vi "t_KCubeActionEngine(V4).vi"(4 "SerialNumber":string="26004283", 5 "Motors // Simulate":bool, 6 "ChannelNumber":i32, 7 "Settings":T1={"Step Size (mm)"=10.0, "Step Delay (ms)"=0, "Velocity (mm/s)"=0.0, "Acceleration (mm/s^2)"=0.0} {"Step Size (mm)" min=0.00046 format="%.8f"}, 8 "error in":errorcluster, 9 "KCubeStepperControl":refnum<k24>(container), 10 "Action":T2, 11 "Input Position":dbl) -> (0 "error out":errorcluster, 1 "KCubeStepperControl Out":refnum<k24>, 2 "IsSettingsInitialized":bool, 3 "Current Position":dbl)   [LabVIEW 2022 SP3]
uses:
  C:/Users/mnopl/Desktop/Software/mnOPSuite/PRISM/Thorlabs.MotionControl.Controls.dll
  PRISM/Thorlabs.MotionControl.Controls.dll
  ActionEngineEnum(V2).ctl
  C:/Users/mnopl/Desktop/Software/mnOPSuite/PRISM/Thorlabs.MotionControl.KCube.StepperMotorCLI.dll
  PRISM/Thorlabs.MotionControl.KCube.StepperMotorCLI.dll
panel:
  in  "Value":dbl
  out "Simulation Status":string="Connection Open"
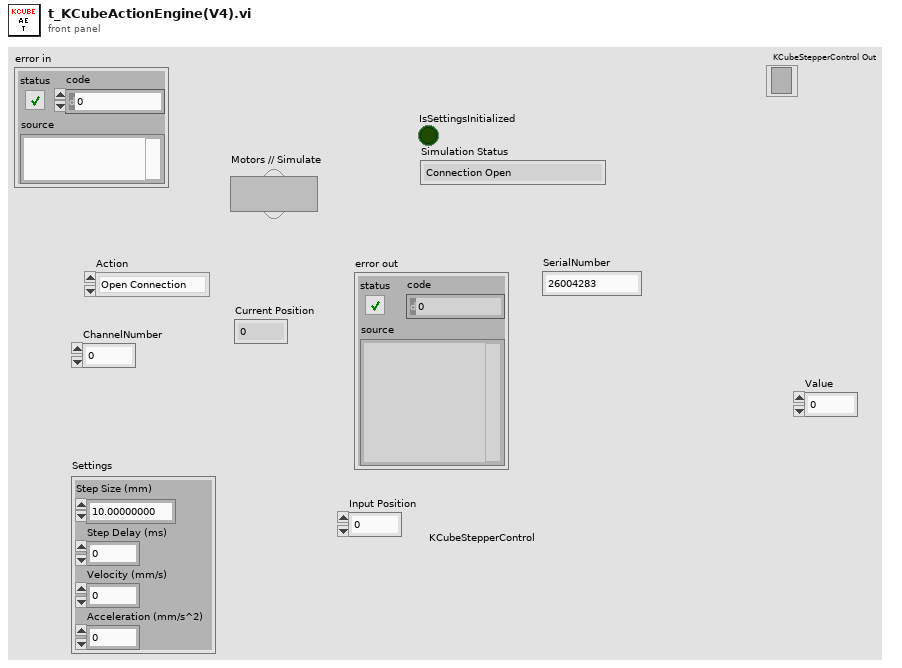
[diagram p1: front panel]
types:
  T1 = cluster{"Step Size (mm)":sgl, "Step Delay (ms)":u32, "Velocity (mm/s)":dbl, "Acceleration (mm/s^2)":dbl}
  T2 = typedef "ActionEngineEnum(V2).ctl" = enum16{"Open Connection", "IsSettingsInitialized? ", "Done", "Get Position", "Settings", "Home", "Move Absolute", "Move Relative", "Step", "Stop Action", "Close Connection"}
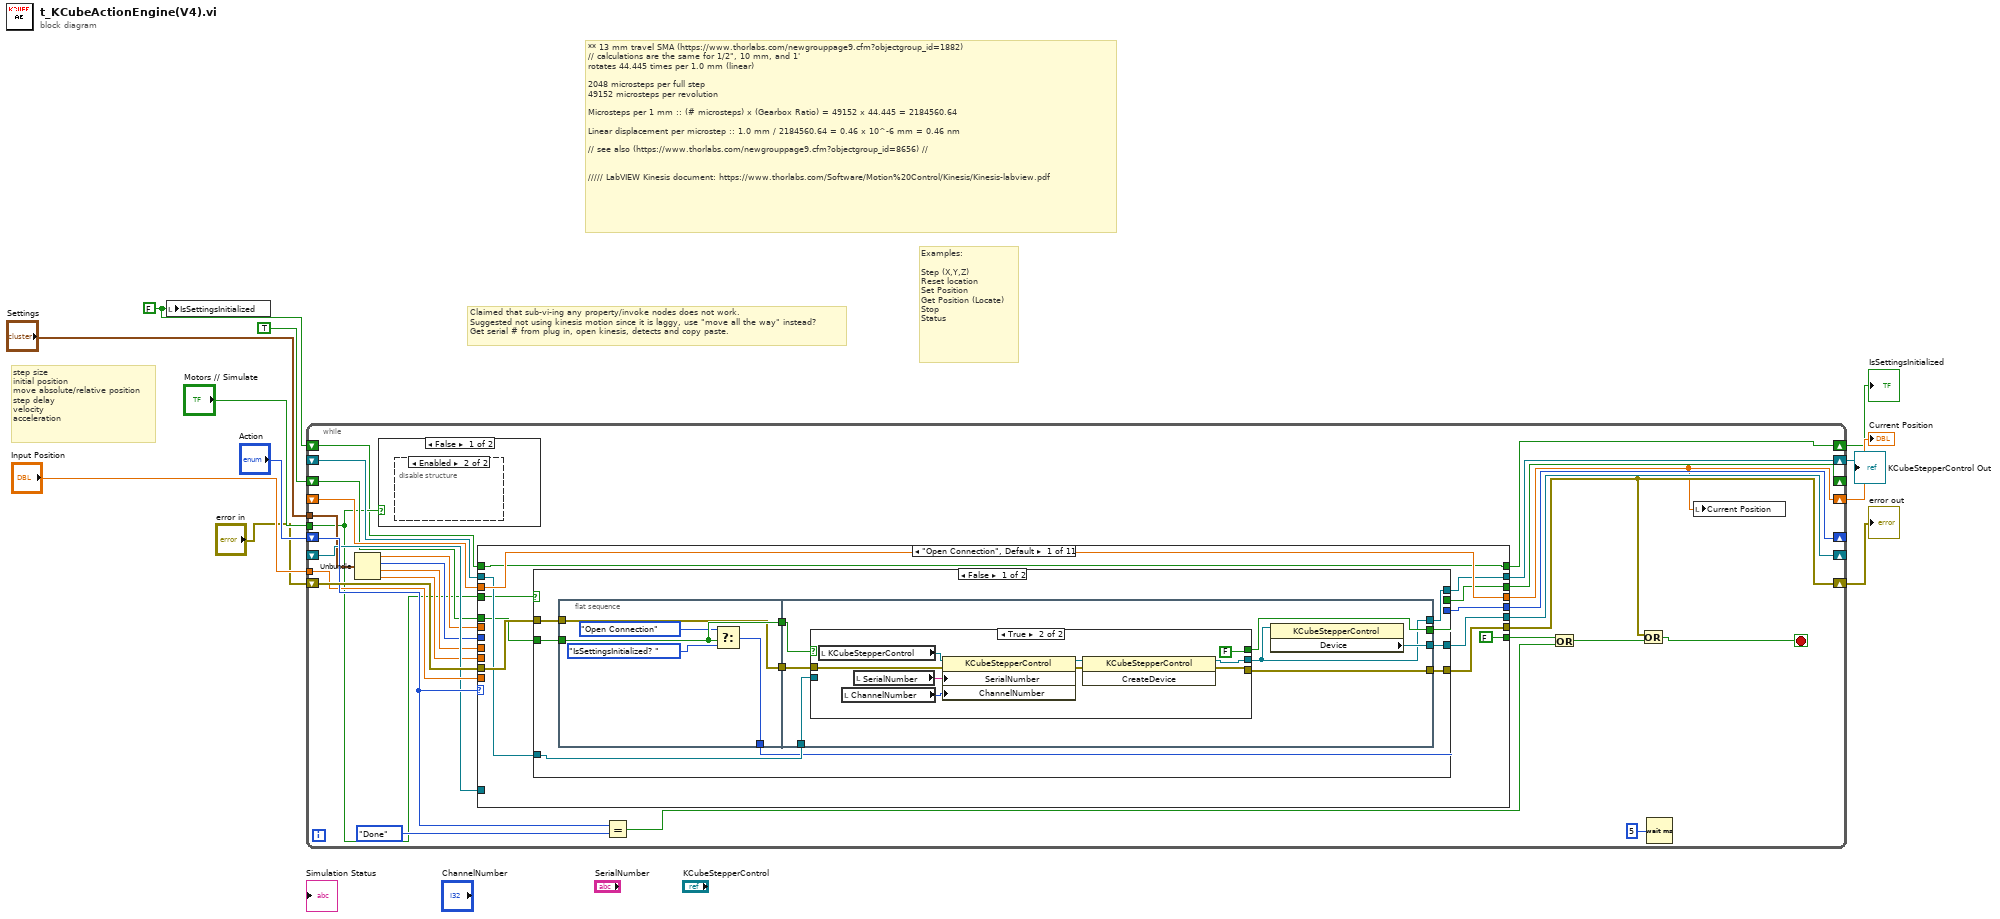
[diagram p0: block diagram]
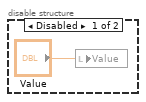
[diagram p2: hidden frame]
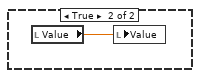
[diagram p3: hidden frame]
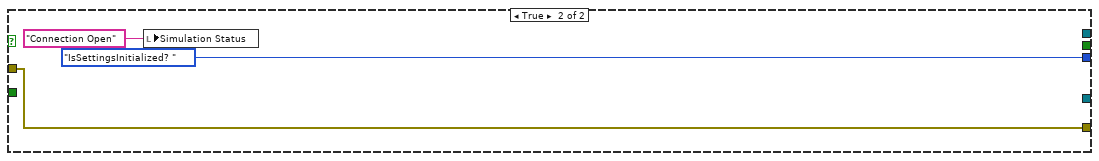
[diagram p5: hidden frame]
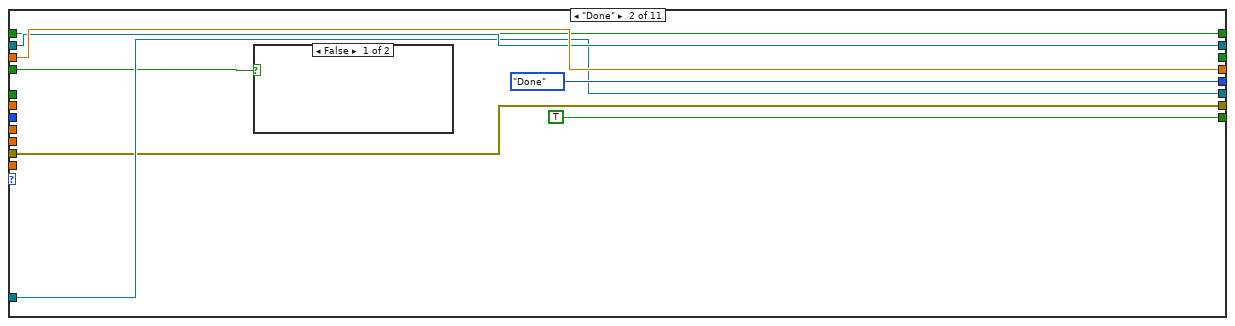
[diagram p6: hidden frame]
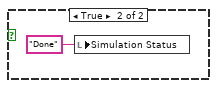
[diagram p7: hidden frame]
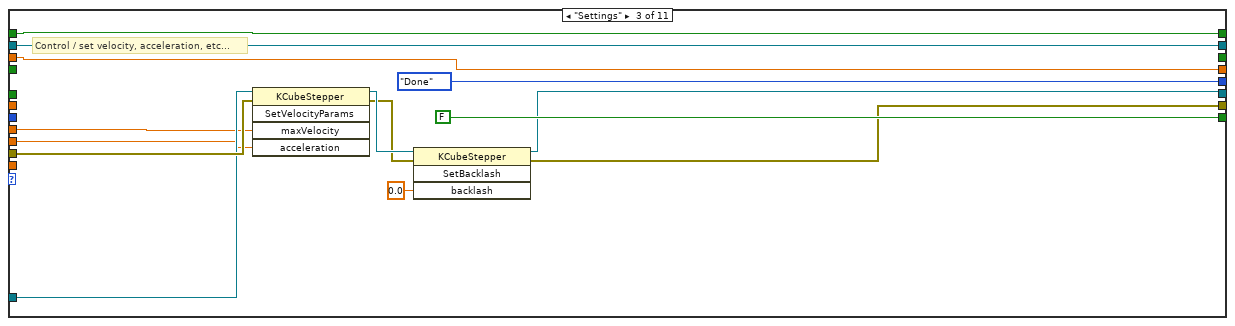
[diagram p8: hidden frame]
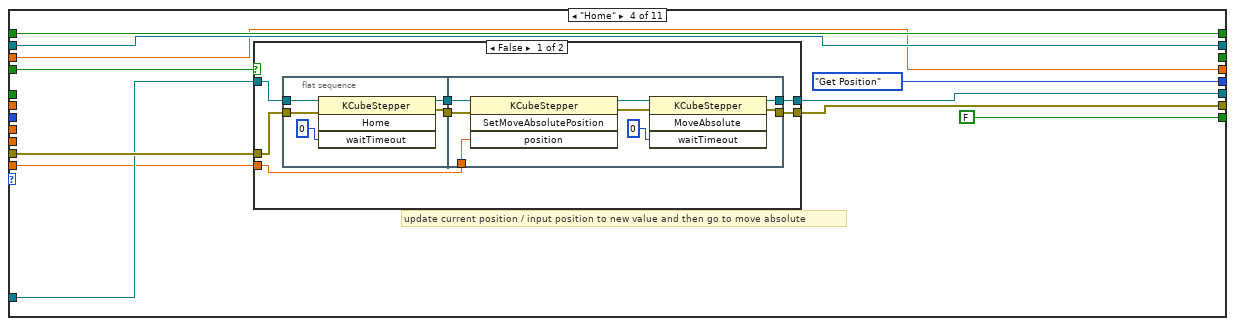
[diagram p9: hidden frame]
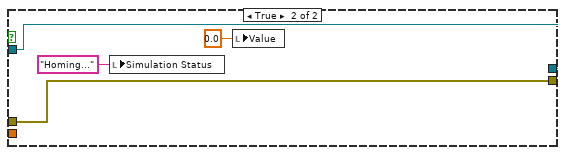
[diagram p10: hidden frame]
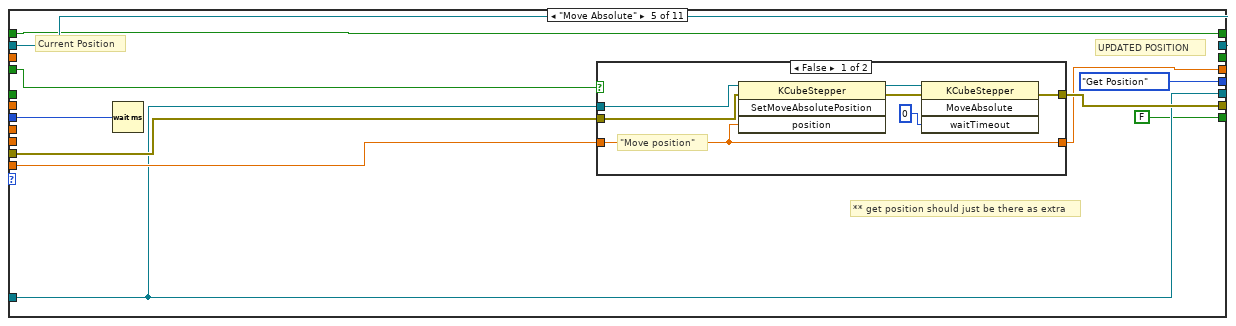
[diagram p11: hidden frame]
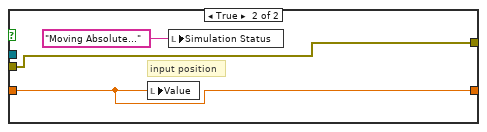
[diagram p12: hidden frame]
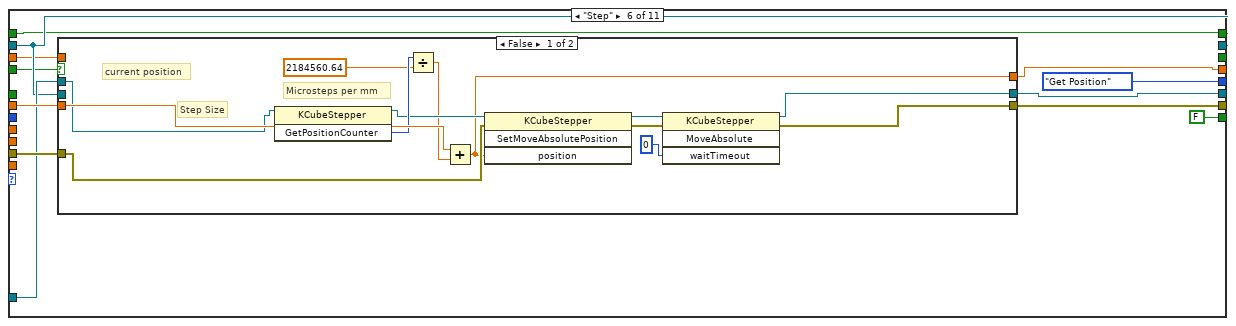
[diagram p13: hidden frame]
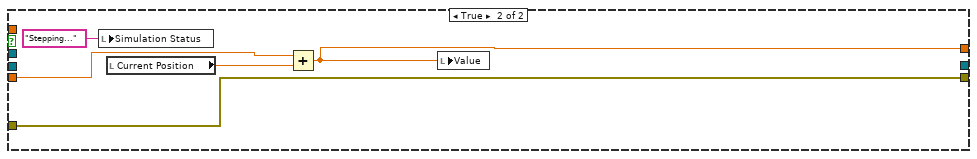
[diagram p14: hidden frame]
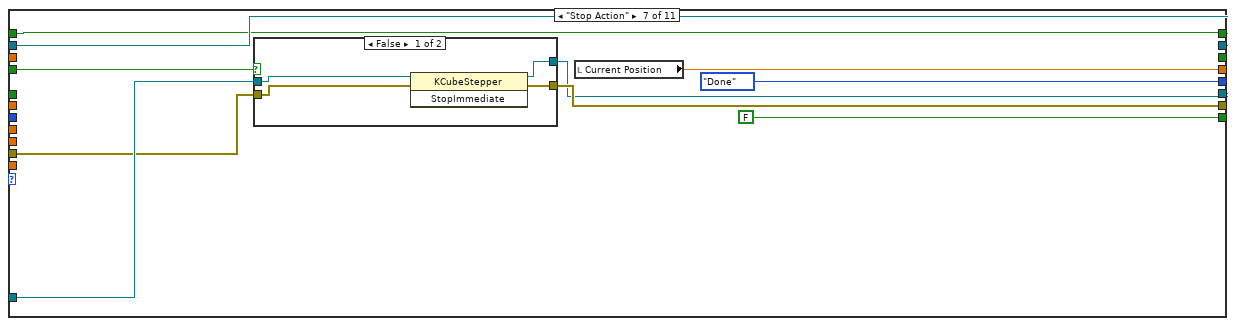
[diagram p15: hidden frame]
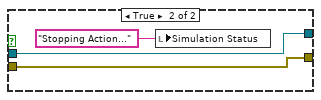
[diagram p16: hidden frame]
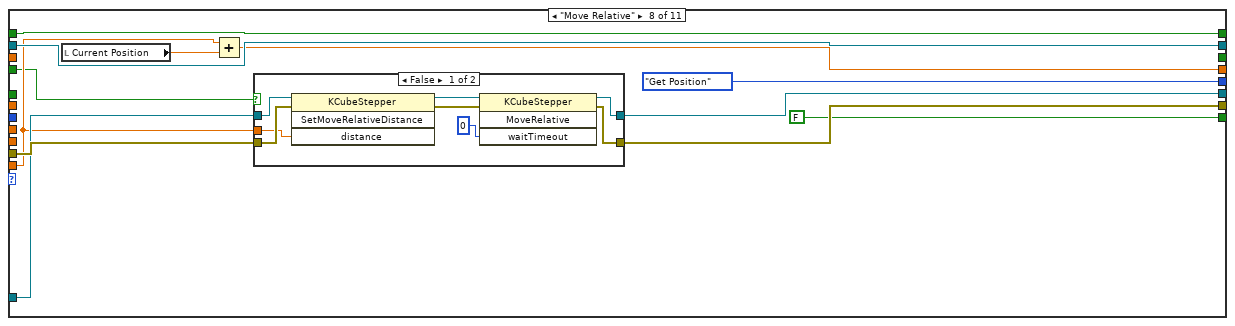
[diagram p17: hidden frame]
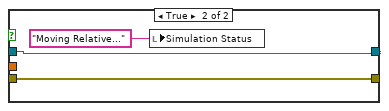
[diagram p18: hidden frame]
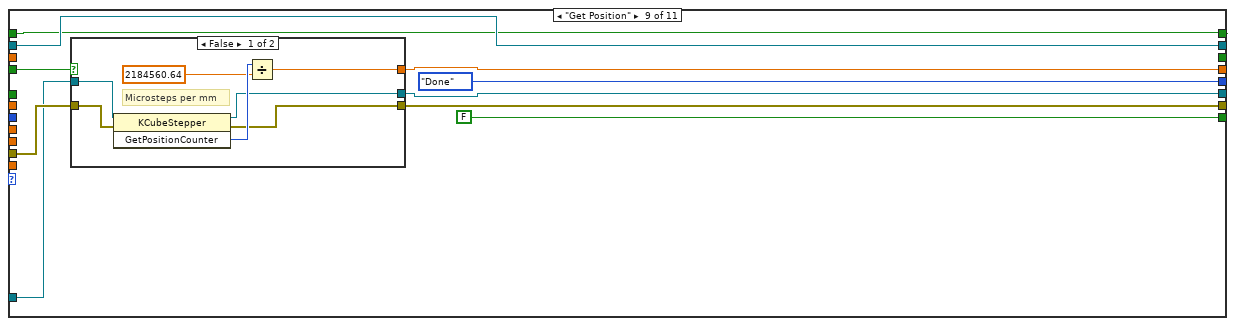
[diagram p19: hidden frame]
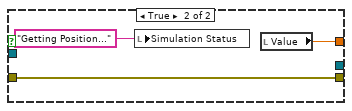
[diagram p20: hidden frame]
diagram:
  w3 = FALSE ("IsSettingsInitialized")
  # "step size\ninitial position\nmove absolute/relative position\nstep delay\nvelocity\nacceleration"
  # "Claimed that sub-vi-ing any property/invoke nodes does not work.\nSuggested not using kinesis motion since it is laggy, use \"move all the way\" instead?\nGet serial # from plug in, open kinesis, detects and copy paste."
  # "Examples:\n\nStep (X,Y,Z)\nReset location\nSet Position\nGet Position (Locate) \nStop\nStatus"
  # "** 13 mm travel SMA (https://www.thorlabs.com/newgrouppage9.cfm?objectgroup_id=1882)\n// calculations are the same for 1/2\", 10 mm, and 1'\nrotates 44.445 times per 1.0 mm (linear)\n\n2048 microsteps per full step\n49152 microsteps per revolution\n\nMicrosteps per 1 mm :: (# microsteps) x (Gearbox Ratio) = 49152 x 44.445 = 2184560.64\n\nLinear displacement per microstep :: 1.0 mm / 2184560.64 = 0.46 x 10^-6 mm = 0.46 nm\n\n// see also (https://www.thorlabs.com/newgrouppage9.cfm?objectgroup_id=8656) //\n\n\n///// LabVIEW Kinesis document: https://www.thorlabs.com/Software/Motion%20Control/Kinesis/Kinesis-labview.pdf"
  n1 = local write "IsSettingsInitialized"(w3) -> ()
  n2 = while {
    shift-right: [w30] -> w11
    shift-left: "error in" -> [w38]
    shift-right: [w36] -> w1
    shift-left: _ -> [w37]
    shift-right: [w34] -> _
    shift-left: "Action" -> [w35]
    tunnel: "Input Position" -> [w32]
    shift-right: [w12] -> w10
    shift-left: _ -> [w31]
    shift-right: [w23] -> _
    shift-left: _ -> [w29]
    shift-right: [w27] -> _
    shift-left: TRUE -> [w28]
    tunnel: "Settings" -> [w22]
    tunnel: "Motors // Simulate" -> [w16]
    shift-right: [w14] -> w4
    shift-left: w3 -> [w13]
    stop <- w15 stop-if-true
    n3 = Unbundle(w22) -> ("Step Size (mm)"=w21:sgl, "Step Delay (ms)"=w20:u32, "Velocity (mm/s)"=w19:dbl, "Acceleration (mm/s^2)"=w18:dbl)
    n4 = case shown="False" w16 {
      frame False {
        n5 = disable-structure shown="Enabled" {
          frame Disabled {
            n6 = local write "Value"("Value") -> ()
          }
          frame Enabled {
          }
        }
      }
      frame True {
        n7 = local read "Value"() -> (w40:dbl)
        n8 = local write "Value"(w40) -> ()
      }
    }
    n9 = case shown="\"Open Connection\", Default" w35 {
      tunnel: w38 -> [w51 w93 w110 w121 w153 w180 w207 w227 w247 w265 w285]
      tunnel: [w48 w93 w99 w122 w156 w179 w205 w226 w246 w263 w284] -> w30
      tunnel: w37 -> [w50 w95 w106 w123 w158 w173 w206 w222 w248 w266 w282]
      tunnel: [w46 w95 w106 w123 w158 w173 w206 w222 w248 w264 w282] -> w36
      tunnel: [w47 ActionEngineEnum(V2)."Done" ("Action") ActionEngineEnum(V2)."Done" ("Enum") ActionEngineEnum(V2)."Get Position" ("Enum") ActionEngineEnum(V2)."Get Position" ("Enum") ActionEngineEnum(V2)."Get Position" ("Enum") ActionEngineEnum(V2)."Done" ("Enum") ActionEngineEnum(V2)."Get Position" ("Enum") ActionEngineEnum(V2)."Done" ("Enum") ActionEngineEnum(V2)."Done" ("Enum") ActionEngineEnum(V2)."Get Position" ("Enum")] -> w34
      tunnel: w21 -> [_ _ _ _ _ w178 _ _ _ _ _]
      tunnel: w32 -> [_ _ _ w117 w157 _ _ w220 _ _ _]
      tunnel: [w52 w97 w112 w113 w148 w177 w203 w221 w244 w267 w281] -> w12
      tunnel: w31 -> [w52 w97 w112 w113 _ w169 _ _ _ w267 w281]
      tunnel: [w45 w94 w101 w119 w152 w175 w204 w223 w242 w262 w286] -> w23
      tunnel: w29 -> [_ w94 w109 w120 w152 w174 w208 w224 w243 _ w287]
      tunnel: w28 -> [w49 _ _ _ _ _ _ _ _ _ _]
      tunnel: [w44 _ _ _ _ _ _ _ _ _ _] -> w27
      tunnel: w20 -> [_ _ _ _ w154 _ _ _ _ _ _]
      tunnel: w19 -> [_ _ w108 _ _ _ _ _ _ _ _]
      tunnel: w18 -> [_ _ w107 _ _ _ _ _ _ _ _]
      tunnel: [w41 w90 w104 w114 w149 w170 w199 w216 w239 w259 w278] -> w14
      tunnel: w16 -> [w43 w91 _ w116 w151 w172 w201 w218 w241 w261 w280]
      tunnel: [FALSE TRUE FALSE FALSE FALSE FALSE FALSE FALSE FALSE FALSE FALSE] -> w17
      tunnel: w13 -> [w41 w90 w104 w114 w149 w170 w199 w216 w239 w259 _]
      frame "Open Connection", Default {
        n10 = case shown="False" w43 {
          tunnel: w51 -> [w60 w89]
          tunnel: w50 -> [w59 _]
          tunnel: w49 -> [w58 _]
          tunnel: [w57 w89] -> w48
          tunnel: [w56 ActionEngineEnum(V2)."IsSettingsInitialized? " ("Enum")] -> w47
          tunnel: [w55 _] -> w46
          tunnel: [w54 _] -> w45
          tunnel: [w53 _] -> w44
          frame False {
            n11 = flat-sequence {
              tunnel: w58 -> [w67]
              tunnel: w60 -> [w64]
              tunnel: [w64] -> w62
              tunnel: [w67] -> w61
              tunnel: [w63] -> w56
              tunnel: w59 -> [w74]
              tunnel: [w69] -> w54
              tunnel: [w73] -> w57
              tunnel: [w68] -> w55
              tunnel: w62 -> [w72]
              tunnel: [w71] -> w53
              tunnel: w61 -> [w70]
              frame #0 {
                n12 = Select(t=ActionEngineEnum(V2)."Open Connection" ("Enum"), s=w67, f=ActionEngineEnum(V2)."IsSettingsInitialized? " ("Enum")) -> (s? t:f=w63:T2)
              }
              frame #1 {
                n13 = case shown="True" w70 {
                  selector: w70 -> [w75 _]
                  tunnel: [w77 w84] -> w73
                  tunnel: w72 -> [w77 w86]
                  tunnel: [w76 w85] -> w68
                  tunnel: w74 -> [w76 _]
                  tunnel: [w75 FALSE] -> w71
                  frame False {
                  }
                  frame True {
                    n14 = local read "KCubeStepperControl"() -> (w81:refnum<k24>)
                    n15 = local read "ChannelNumber"() -> (w78:i32)
                    n16 = local read "SerialNumber"() -> (w80:string)
                    n17 = property class="KCubeStepperControl"(reference=w81, error in=w86, "SerialNumber"=w80, "ChannelNumber"=w78) -> (reference out=w83:refnum<k24>, error out=w82:errorcluster)
                    n18 = invoke class="KCubeStepperControl" method="CreateDevice"(reference=w83, error in=w82) -> (reference out=w85:refnum<k24>, error out=w84:errorcluster)  [unwired: 1 in, 1 out]
                  }
                }
                n19 = property class="KCubeStepperControl"(reference=w68) -> ("Device"=w69:refnum<k24>)  [unwired: 1 in, 2 out]
              }
            }
          }
          frame True {
            n20 = local write "Simulation Status"("Connection Open") -> ()
          }
        }
      }
      frame "Done" {
        n21 = case shown="False" w91 {
          frame False {
          }
          frame True {
            n22 = local write "Simulation Status"("Done" ("Status")) -> ()
          }
        }
      }
      frame "Settings" {
        # "Control / set velocity, acceleration, etc..."
        n23 = invoke class="KCubeStepper" method="SetVelocityParams"(reference=w109, error in=w110, "maxVelocity"=w108, "acceleration"=w107) -> (reference out=w102:refnum<k24>, error out=w100:errorcluster)  [unwired: 1 in, 3 out]
        n24 = invoke class="KCubeStepper" method="SetBacklash"(reference=w102, error in=w100, "backlash"=0.0) -> (reference out=w101:refnum<k24>, error out=w99:errorcluster)  [unwired: 1 in, 2 out]
      }
      frame "Home" {
        # "update current position / input position to new value and then go to move absolute"
        n25 = case shown="False" w116 {
          tunnel: [w128 w145] -> w122
          tunnel: w121 -> [w127 w145]
          tunnel: w120 -> [w126 w144]
          tunnel: [w125 w144] -> w119
          tunnel: w117 -> [w124 _]
          frame False {
            n26 = flat-sequence {
              tunnel: w126 -> [w135]
              tunnel: w127 -> [w133]
              tunnel: [w132] -> w130
              tunnel: [w131] -> w129
              tunnel: w130 -> [w143]
              tunnel: w129 -> [w142]
              tunnel: [w138] -> w128
              tunnel: w124 -> [w137]
              tunnel: [w136] -> w125
              frame #0 {
                n27 = invoke class="KCubeStepper" method="Home"(reference=w135, error in=w133, "waitTimeout"=0) -> (reference out=w132:refnum<k24>, error out=w131:errorcluster)  [unwired: 1 in, 2 out]
              }
              frame #1 {
                n28 = invoke class="KCubeStepper" method="SetMoveAbsolutePosition"(reference=w143, error in=w142, "position"=w137) -> (reference out=w140:refnum<k24>, error out=w141:errorcluster)  [unwired: 1 in, 2 out]
                n29 = invoke class="KCubeStepper" method="MoveAbsolute"(reference=w140, error in=w141, "waitTimeout"=0) -> (reference out=w136:refnum<k24>, error out=w138:errorcluster)  [unwired: 1 in, 2 out]
              }
            }
          }
          frame True {
            n30 = local write "Simulation Status"("Homing..." ("Simulation Status")) -> ()
            n31 = local write "Value"(0.0 ("Value")) -> ()
          }
        }
      }
      frame "Move Absolute" {
        # "** get position should just be there as extra"
        # "UPDATED POSITION"
        # "Current Position"
        n32 = Wait (ms)(milliseconds to wait=w154) -> ()  [unwired: 1 out]
        n33 = case shown="False" w151 {
          tunnel: w157 -> [w159 w166]
          tunnel: [w165 w168] -> w156
          tunnel: w153 -> [w164 w168]
          tunnel: w152 -> [w163 _]
          tunnel: [w159 w166] -> w148
          frame False {
            # "\"Move position\""
            n34 = invoke class="KCubeStepper" method="SetMoveAbsolutePosition"(reference=w163, error in=w164, "position"=w159) -> (reference out=w161:refnum<k24>, error out=w162:errorcluster)  [unwired: 1 in, 2 out]
            n35 = invoke class="KCubeStepper" method="MoveAbsolute"(reference=w161, error in=w162, "waitTimeout"=0) -> (error out=w165:errorcluster)  [unwired: 1 in, 3 out]
          }
          frame True {
            # "input position"
            n36 = local write "Value"(w166) -> ()
            n37 = local write "Simulation Status"("Moving Absolute..." ("Status")) -> ()
          }
        }
      }
      frame "Step" {
        n38 = case shown="False" w172 {
          tunnel: w180 -> [w190 w198]
          tunnel: [w189 w198] -> w179
          tunnel: w178 -> [w188 w197]
          tunnel: [w181 w195] -> w177
          tunnel: [w187 _] -> w175
          tunnel: w174 -> [w184 _]
          tunnel: w173 -> [_ _]
          tunnel: w169 -> [_ _]
          frame False {
            # "Microsteps per mm"
            # "current position"
            # "Step Size"
            n39 = invoke class="KCubeStepper" method="GetPositionCounter"(reference=w184) -> (reference out=w183:refnum<k24>, "GetPositionCounter"=w186:i32)  [unwired: 2 in, 1 out]
            n40 = Divide(x=w186, y=2184560.64) -> (x/y=w182:dbl)
            n41 = Add(x=w188, y=w182) -> (x+y=w181:dbl)
            n42 = invoke class="KCubeStepper" method="SetMoveAbsolutePosition"(reference=w183, error in=w190, "position"=w181) -> (reference out=w192:refnum<k24>, error out=w193:errorcluster)  [unwired: 1 in, 2 out]
            n43 = invoke class="KCubeStepper" method="MoveAbsolute"(reference=w192, error in=w193, "waitTimeout"=0) -> (reference out=w187:refnum<k24>, error out=w189:errorcluster)  [unwired: 1 in, 2 out]
          }
          frame True {
            n44 = local write "Simulation Status"("Stepping..." ("Simulation Status")) -> ()
            n45 = local read "Current Position"() -> (w196:dbl)
            n46 = Add(x=w197, y=w196) -> (x+y=w195:dbl)
            n47 = local write "Value"(w195) -> ()
          }
        }
      }
      frame "Stop Action" {
        n48 = case shown="False" w201 {
          tunnel: w208 -> [w212 w213]
          tunnel: w207 -> [w211 w214]
          tunnel: [w210 w214] -> w205
          tunnel: [w209 w213] -> w204
          frame False {
            n49 = invoke class="KCubeStepper" method="StopImmediate"(reference=w212, error in=w211) -> (reference out=w209:refnum<k24>, error out=w210:errorcluster)  [unwired: 1 in, 1 out]
          }
          frame True {
            n50 = local write "Simulation Status"("Stopping Action..." ("Simulation Status")) -> ()
          }
        }
        n51 = local read "Current Position"() -> (w203:dbl)
      }
      frame "Move Relative" {
        n52 = local read "Current Position"() -> (w219:dbl)
        n53 = Add(x=w220, y=w219) -> (x+y=w221:dbl)
        n54 = case shown="False" w218 {
          tunnel: w227 -> [w232 w237]
          tunnel: [w231 w237] -> w226
          tunnel: w224 -> [w230 w238]
          tunnel: [w229 w238] -> w223
          tunnel: w220 -> [w228 _]
          frame False {
            n55 = invoke class="KCubeStepper" method="SetMoveRelativeDistance"(reference=w230, error in=w232, "distance"=w228) -> (reference out=w234:refnum<k24>, error out=w235:errorcluster)  [unwired: 1 in, 2 out]
            n56 = invoke class="KCubeStepper" method="MoveRelative"(reference=w234, error in=w235, "waitTimeout"=0) -> (reference out=w229:refnum<k24>, error out=w231:errorcluster)  [unwired: 1 in, 2 out]
          }
          frame True {
            n57 = local write "Simulation Status"("Moving Relative..." ("Simulation Status")) -> ()
          }
        }
      }
      frame "Get Position" {
        n58 = case shown="False" w241 {
          tunnel: w247 -> [w255 w258]
          tunnel: [w252 w258] -> w246
          tunnel: [w251 w256] -> w244
          tunnel: w243 -> [w250 _]
          tunnel: [w249 _] -> w242
          frame False {
            # "Microsteps per mm"
            n59 = invoke class="KCubeStepper" method="GetPositionCounter"(reference=w250, error in=w255) -> (reference out=w249:refnum<k24>, error out=w252:errorcluster, "GetPositionCounter"=w254:i32)  [unwired: 1 in]
            n60 = Divide(x=w254, y=2184560.64) -> (x/y=w251:dbl)
          }
          frame True {
            n61 = local write "Simulation Status"("Getting Position..." ("Status")) -> ()
            n62 = local read "Value"() -> (w256:dbl)
          }
        }
      }
      frame "Close Connection" {
        # "DEVICE Output"
        n63 = case shown="False" w261 {
          tunnel: w266 -> [w275 _]
          tunnel: w265 -> [w274 w276]
          tunnel: [w273 _] -> w264
          tunnel: [w272 w276] -> w263
          tunnel: [w269 _] -> w262
          frame False {
            n64 = property class="KCubeStepperControl"(reference=w275) -> (reference out=w271:refnum<k24>, "Device"=w270:refnum<k24>)  [unwired: 1 in, 1 out]
            n65 = invoke class="KCubeStepperControl" method="CloseDevice"(reference=w271, error in=w274) -> (reference out=w273:refnum<k24>, error out=w272:errorcluster)  [unwired: 1 in, 1 out]
            n66 = invoke class="KCubeStepper" method="Disconnect"(reference=w270) -> (reference out=w269:refnum<k24>)  [unwired: 2 in, 2 out]
          }
          frame True {
            n67 = local write "Simulation Status"("Closing Connection..." ("Simulation Status")) -> ()
          }
        }
      }
      frame "IsSettingsInitialized? " {
        n68 = case shown="True" w280 {
          tunnel: w287 -> [w292 _]
          tunnel: [w291 _] -> w286
          tunnel: w285 -> [w290 w295]
          tunnel: [w289 w295] -> w284
          tunnel: [w288 TRUE] -> w278
          frame False {
            n69 = invoke class="KCubeStepper" method="IsSettingsInitialized"(reference=w292, error in=w290) -> (reference out=w291:refnum<k24>, error out=w289:errorcluster, "IsSettingsInitialized"=w288:bool)  [unwired: 1 in]
          }
          frame True {
            n70 = local write "Simulation Status"("Settings Initialized" ("Status")) -> ()
          }
        }
      }
    }
    n71 = Equal?(x=w35, y=ActionEngineEnum(V2)."Done" ("Enum")) -> (x = y?=w25:bool)
    n72 = Or(x=w17, y=w25) -> (x .or. y?=w26:bool)
    n73 = Or(x=w30, y=w26) -> (x .or. y?=w15:bool)
    n74 = Wait (ms)(milliseconds to wait=u32 5) -> ()  [unwired: 1 out]
    n75 = local write "Current Position"(w12) -> ()
  }
  "error out" <- w11
  "Current Position" <- w10
  "IsSettingsInitialized" <- w4
  "KCubeStepperControl Out" <- w1
